vi "_089.vi"() -> ()   [LabVIEW 2024]
panel:
  out "o/p":dbl
  out "o/p":dbl[](array[numeric])
  out "o/p":dbl[](array[numeric])
  # "Fundamentals :"
  # "18~>After running this VI,what is the value displayed in the o/p & iteration count?"
  # "Nrml Approach :"
  # "Dfrnt Approach :"
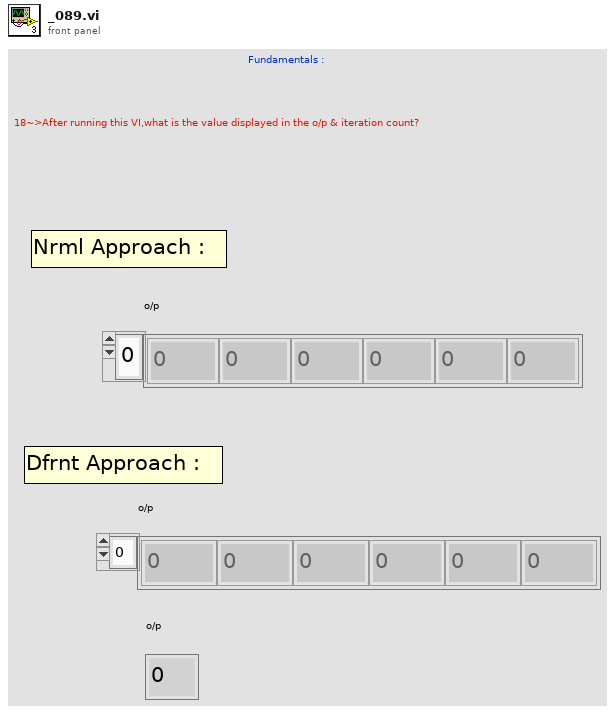
[diagram p1: front panel]
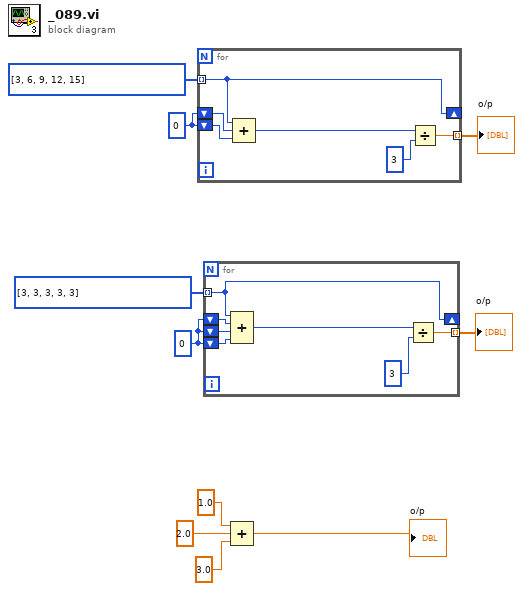
[diagram p0: block diagram]
diagram:
  w5 = 0
  w10 = 0
  n1 = for {
    shift-right: [w11] -> _
    shift-left: w10 -> [w16]
    shift-left: w10 -> [w15]
    tunnel: [w12] -> w9 mode=indexing
    tunnel: i32[] [3, 6, 9, 12, 15] -> [w11] mode=indexing
    n2 = Compound Arithmetic op=ADD(w11, w16, w15) -> (w14:i32)
    n3 = Divide(x=w14, y=3) -> (x/y=w12:dbl)
  }
  "o/p" <- w9
  n4 = for {
    shift-right: [w18] -> _
    shift-left: w5 -> [w23]
    shift-left: w5 -> [w22]
    tunnel: [w19] -> w6 mode=indexing
    tunnel: i32[] [3, 3, 3, 3, 3] -> [w18] mode=indexing
    shift-left: w5 -> [w17]
    n5 = Compound Arithmetic op=ADD(w18, w23, w22, w17) -> (w21:i32)
    n6 = Divide(x=w21, y=3) -> (x/y=w19:dbl)
  }
  "o/p" <- w6
  n7 = Compound Arithmetic op=unknown(1.0 ("value"), 2.0 ("value"), 3.0 ("value")) -> (→"o/p":dbl)
